vi "digital_lowpass.vi"() -> ()   [LabVIEW 2023]
uses:
  <vilib>/addons/Biomedical/Biosignal Measurements/EEG/EEG FFT Spectrum (Waveform).vi
  <vilib>/addons/Biomedical/NI_BMTK_Measurements.lvlib
panel:
  out "EEG FFT Spectrum before filtering":cluster{"f0":dbl, "df":dbl, "S(f)":dbl[]}(graph)
  out "EEG Signal":dynamicdata(graph)
  out "Gamma Wave FFT Spectrum":cluster{"f0":dbl, "df":dbl, "S(f)":dbl[]}(graph)
  out "Beta Wave FFT Spectrum":cluster{"f0":dbl, "df":dbl, "S(f)":dbl[]}(graph)
  out "Alpha Wave FFT Spectrum":cluster{"f0":dbl, "df":dbl, "S(f)":dbl[]}(graph)
  out "Theta Wave FFT Spectrum":cluster{"f0":dbl, "df":dbl, "S(f)":dbl[]}(graph)
  out "Delta Wave FFT Spectrum":cluster{"f0":dbl, "df":dbl, "S(f)":dbl[]}(graph)
  out "FFT Spectrum":cluster{"f0":dbl, "df":dbl, "S(f)":dbl[]}(graph)
  out "Delta Wave":dynamicdata(graph)
  out "Gamma":dynamicdata(graph)
  out "Beta":dynamicdata(graph)
  out "Alpha Wave":dynamicdata(graph)
  out "Theta Wave":dynamicdata(graph)
  out "After High-pass: fc = 1 Hz":dynamicdata(graph)
  out "After Low-pass: fc = 40 Hz":dynamicdata(graph)
  in  "stop":bool
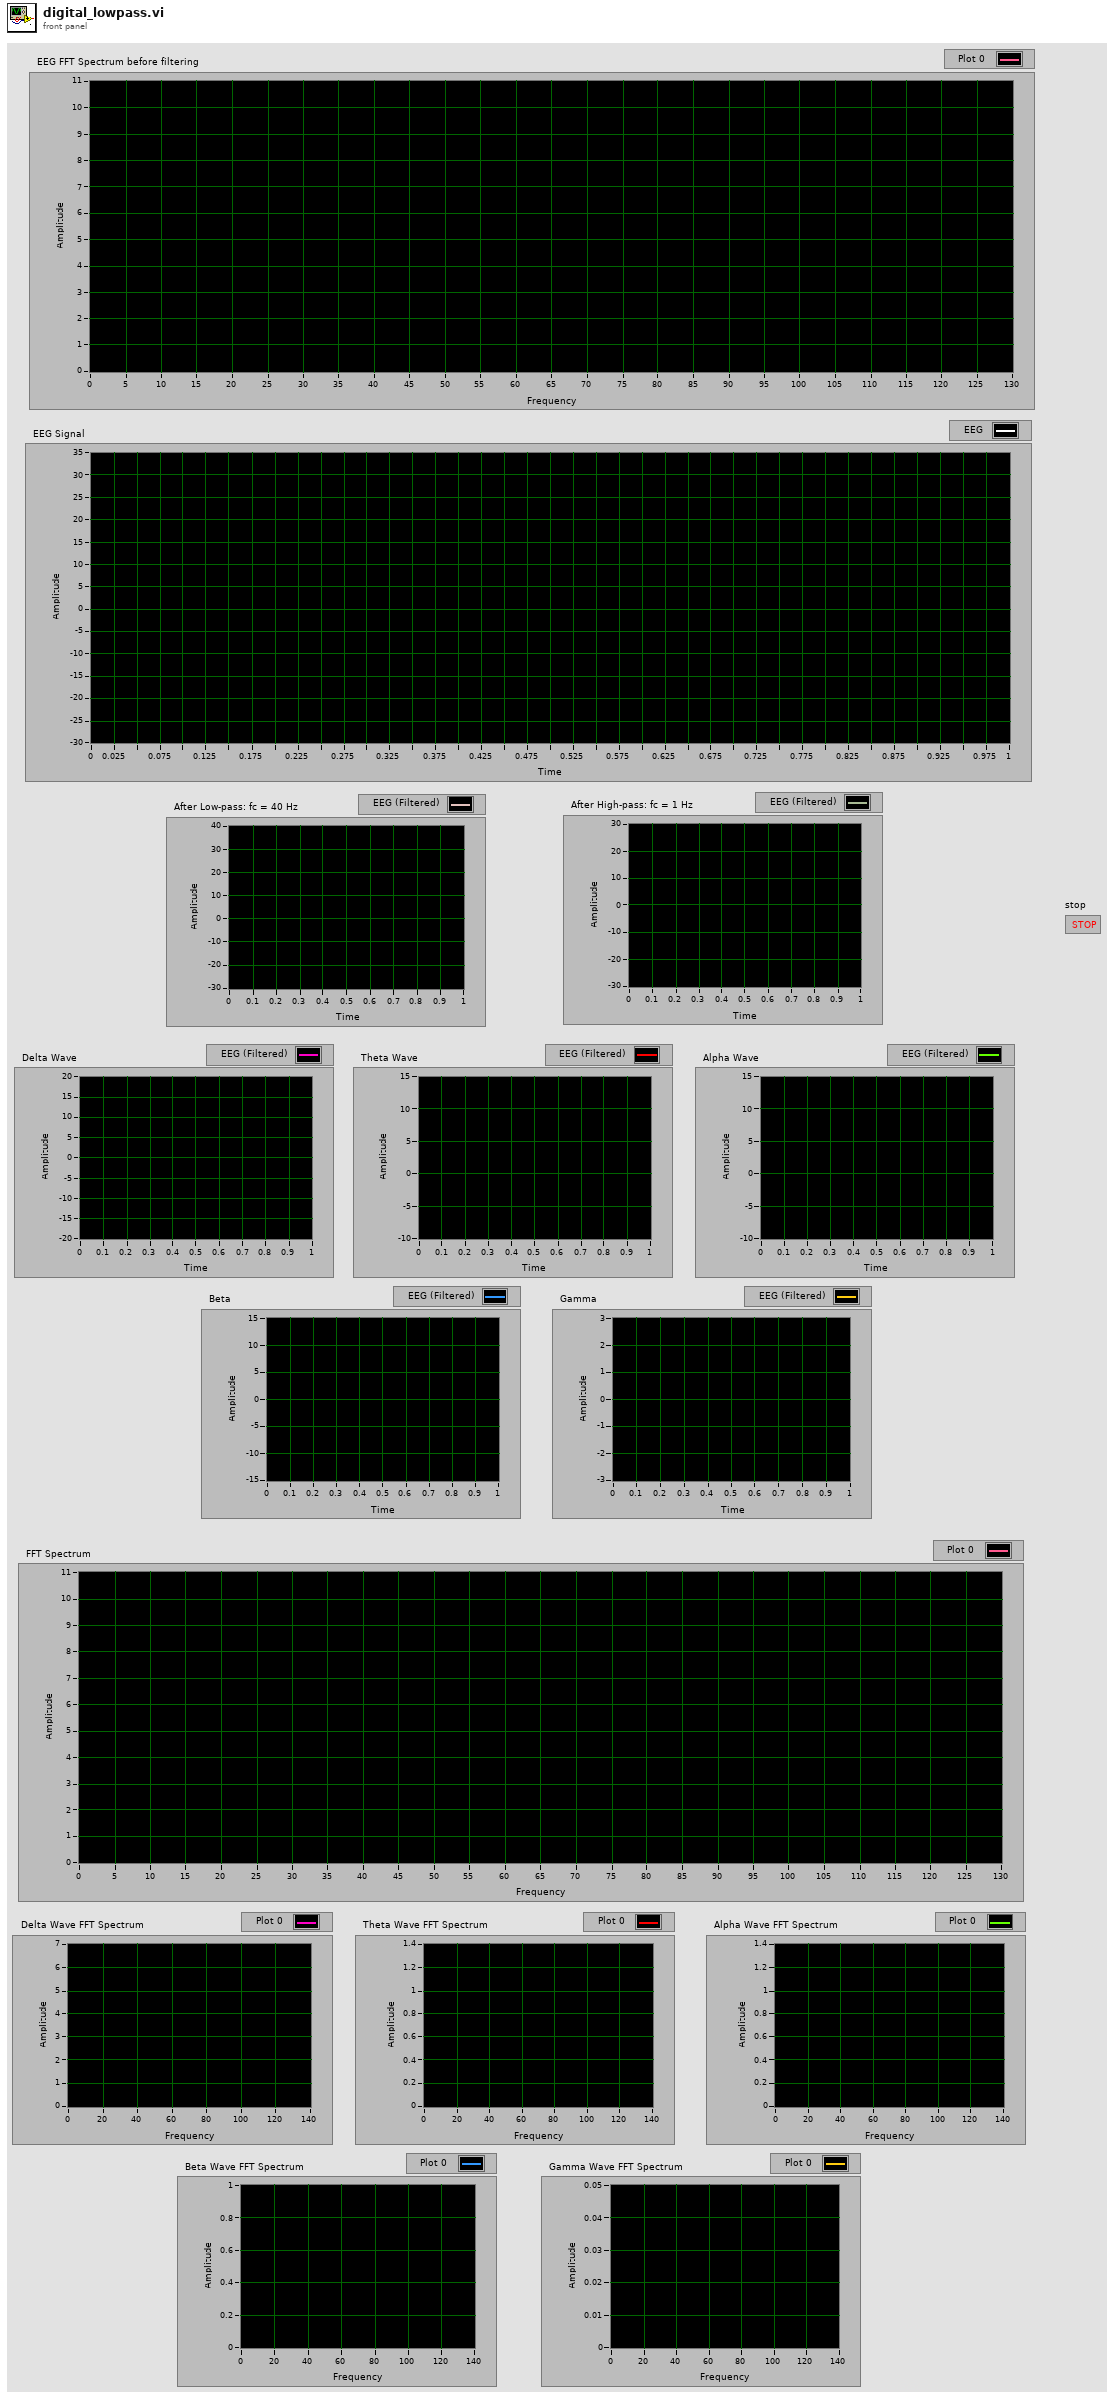
[diagram p1: front panel]
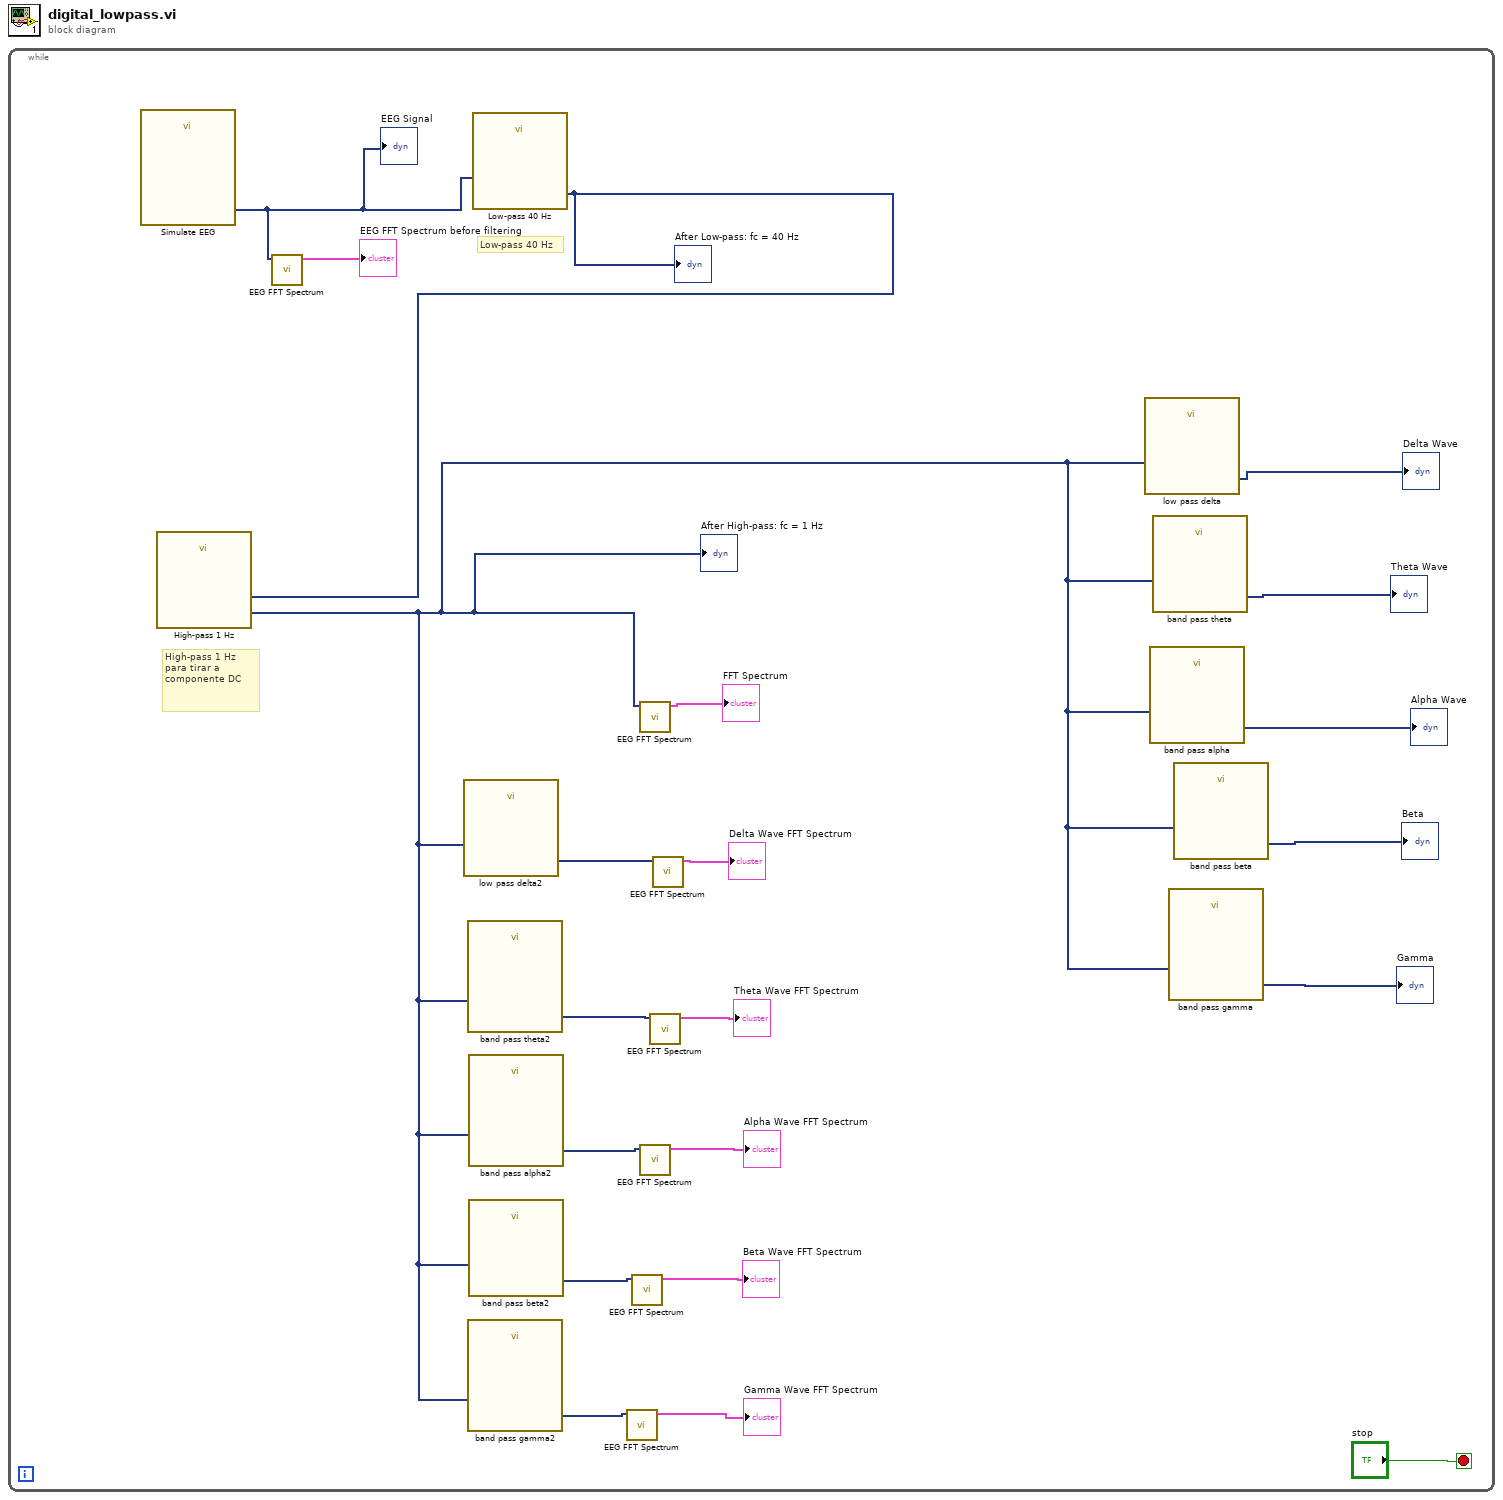
[diagram p0: block diagram]
diagram:
  n1 = while {
    stop <- "stop" stop-if-true
    # "Low-pass 40 Hz"
    # "High-pass 1 Hz para tirar a componente DC"
    n2 = call "Simulate EEG"() -> ("EEG"=w2:dynamicdata)  [unwired: 10 in, 1 out]
    "EEG Signal" <- w2
    n3 = call-poly <vilib>:"EEG FFT Spectrum.vi"("EEG"=w2) -> ("FFT spectrum"=→"EEG FFT Spectrum before filtering":cluster{"f0":dbl, "df":dbl, "S(f)":dbl[]})  [unwired: 8 in, 2 out]
    n4 = call "Low-pass 40 Hz"("Signal"=w2) -> ("Filtered Signal"=w1:dynamicdata)  [unwired: 9 in, 1 out]
    "After Low-pass: fc = 40 Hz" <- w1
    n5 = call "High-pass 1 Hz"("Signal"=w1) -> ("Filtered Signal"=w14:dynamicdata)  [unwired: 9 in, 1 out]
    "After High-pass: fc = 1 Hz" <- w14
    n6 = call "low pass delta2"("Signal"=w14) -> ("Filtered Signal"=w12:dynamicdata)  [unwired: 9 in, 1 out]
    n7 = call "band pass theta2"("Signal"=w14) -> ("Filtered Signal"=w11:dynamicdata)  [unwired: 9 in, 1 out]
    n8 = call "band pass gamma2"("Signal"=w14) -> ("Filtered Signal"=w4:dynamicdata)  [unwired: 9 in, 1 out]
    n9 = call "band pass alpha2"("Signal"=w14) -> ("Filtered Signal"=w8:dynamicdata)  [unwired: 9 in, 1 out]
    n10 = call "band pass beta2"("Signal"=w14) -> ("Filtered Signal"=w6:dynamicdata)  [unwired: 9 in, 1 out]
    n11 = call-poly <vilib>:"EEG FFT Spectrum.vi"("EEG"=w4) -> ("FFT spectrum"=→"Gamma Wave FFT Spectrum":cluster{"f0":dbl, "df":dbl, "S(f)":dbl[]})  [unwired: 8 in, 2 out]
    n12 = call-poly <vilib>:"EEG FFT Spectrum.vi"("EEG"=w6) -> ("FFT spectrum"=→"Beta Wave FFT Spectrum":cluster{"f0":dbl, "df":dbl, "S(f)":dbl[]})  [unwired: 8 in, 2 out]
    n13 = call-poly <vilib>:"EEG FFT Spectrum.vi"("EEG"=w14) -> ("FFT spectrum"=→"FFT Spectrum":cluster{"f0":dbl, "df":dbl, "S(f)":dbl[]})  [unwired: 8 in, 2 out]
    n14 = call-poly <vilib>:"EEG FFT Spectrum.vi"("EEG"=w8) -> ("FFT spectrum"=→"Alpha Wave FFT Spectrum":cluster{"f0":dbl, "df":dbl, "S(f)":dbl[]})  [unwired: 8 in, 2 out]
    n15 = call-poly <vilib>:"EEG FFT Spectrum.vi"("EEG"=w11) -> ("FFT spectrum"=→"Theta Wave FFT Spectrum":cluster{"f0":dbl, "df":dbl, "S(f)":dbl[]})  [unwired: 8 in, 2 out]
    n16 = call-poly <vilib>:"EEG FFT Spectrum.vi"("EEG"=w12) -> ("FFT spectrum"=→"Delta Wave FFT Spectrum":cluster{"f0":dbl, "df":dbl, "S(f)":dbl[]})  [unwired: 8 in, 2 out]
    n17 = call "low pass delta"("Signal"=w14) -> ("Filtered Signal"=→"Delta Wave":dynamicdata)  [unwired: 9 in, 1 out]
    n18 = call "band pass alpha"("Signal"=w14) -> ("Filtered Signal"=→"Alpha Wave":dynamicdata)  [unwired: 9 in, 1 out]
    n19 = call "band pass theta"("Signal"=w14) -> ("Filtered Signal"=→"Theta Wave":dynamicdata)  [unwired: 9 in, 1 out]
    n20 = call "band pass gamma"("Signal"=w14) -> ("Filtered Signal"=→"Gamma":dynamicdata)  [unwired: 9 in, 1 out]
    n21 = call "band pass beta"("Signal"=w14) -> ("Filtered Signal"=→"Beta":dynamicdata)  [unwired: 9 in, 1 out]
  }
